vi "gradient_ascent_test.vi"() -> ()   [LabVIEW 2024]
uses:
  <vilib>/numeric/Random Number (Range) DBL.vi
panel:
  in  "N trials":dbl=16.0
  out "diff":dbl
  out "XY Graph 2":cluster{dbl[], dbl[]}[](graph)
  out "end result":dbl
  in  "k":dbl=150.0
  out "start X":dbl=75.0
  out "StdDev":dbl
  out "Mean":dbl
  # "Used only to create Gaussian to optimize"
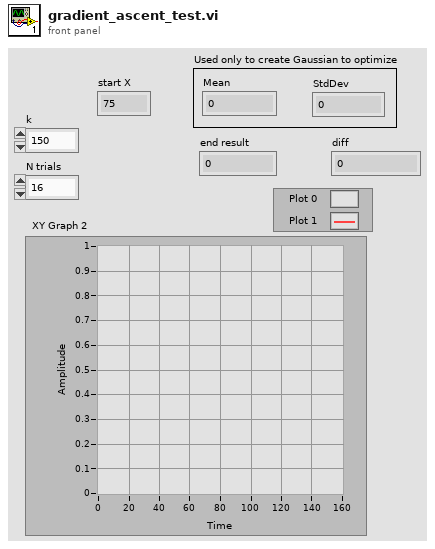
[diagram p1: front panel]
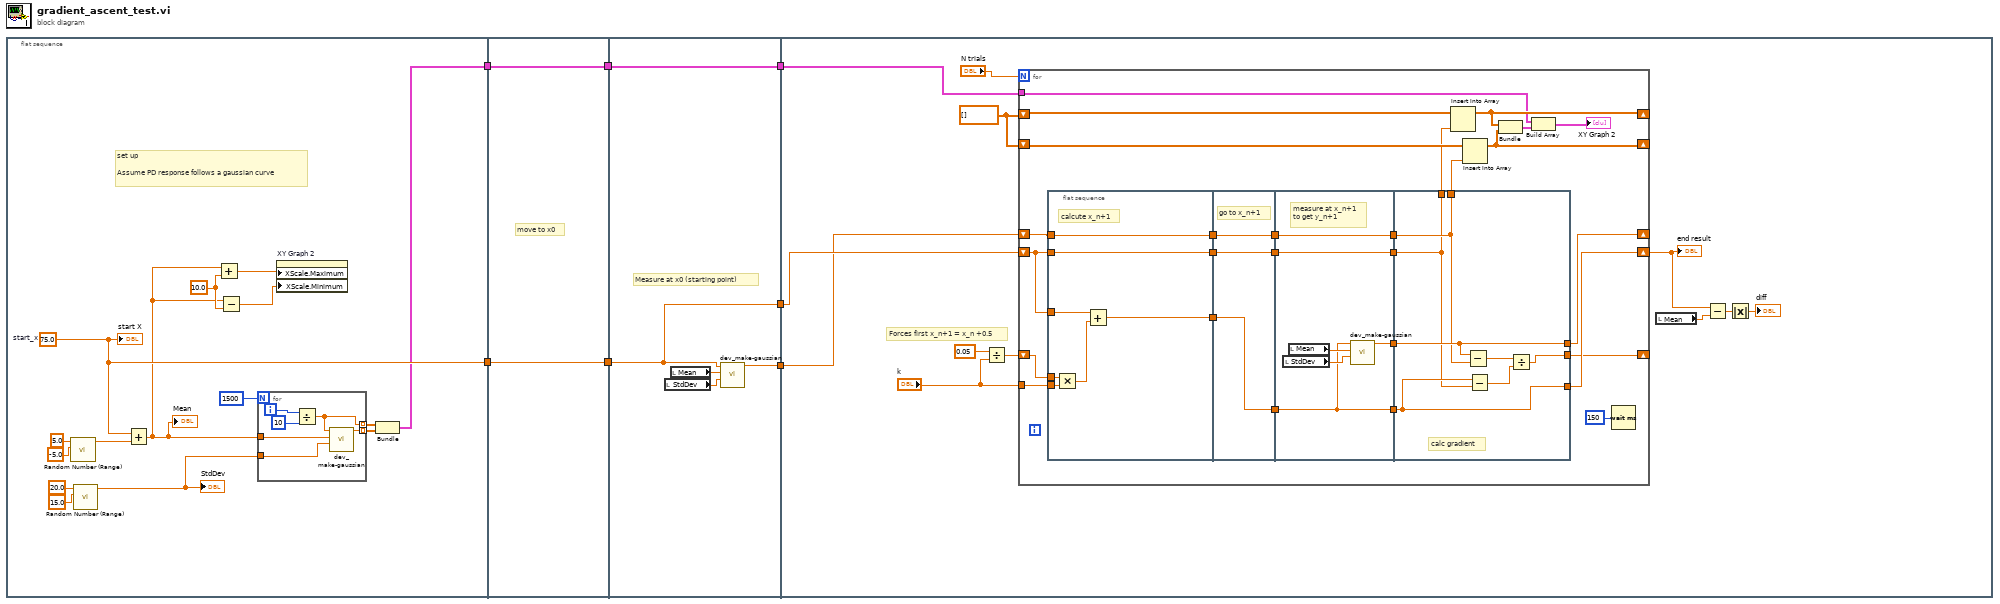
[diagram p0: block diagram]
diagram:
  n1 = flat-sequence {
    tunnel: [w13] -> w7
    tunnel: [w12] -> w1
    tunnel: w7 -> [w30]
    tunnel: [w30] -> w6
    tunnel: [w29] -> w2
    tunnel: w1 -> [w29]
    tunnel: w6 -> [w32]
    tunnel: [w33] -> w5
    tunnel: [w32] -> w4
    tunnel: [w31] -> w3
    tunnel: w2 -> [w31]
    tunnel: w5 -> [w46]
    tunnel: w4 -> [w47]
    tunnel: w3 -> [w40]
    frame #0 {
      w9 = 10.0 ("y")
      w13 = 75.0  # start_x
      # "set up\n\nAssume PD response follows a gaussian curve"
      n2 = call-poly <vilib>:"Random Number (Range).vi"("lower bound (0)"=-5.0, "upper bound (100)"=5.0) -> ("number"=w14:dbl)  [unwired: 9 in]
      n3 = call-poly <vilib>:"Random Number (Range).vi"("lower bound (0)"=15.0, "upper bound (100)"=20.0) -> ("number"=w20:dbl)  [unwired: 9 in]
      "StdDev" <- w20
      n4 = Add(x=w13, y=w14) -> (x+y=w8:dbl)
      "Mean" <- w8
      n5 = Add(x=w8, y=w9) -> (x+y=w11:dbl)
      n6 = Subtract(x=w8, y=w9) -> (x-y=w10:dbl)
      n7 = for {
        N: 1500 -> [_]
        tunnel: w20 -> [w28]
        tunnel: [w27] -> w18 mode=indexing
        tunnel: [w24] -> w17 mode=indexing
        tunnel: w8 -> [w26]
        i -> [w25]
        n8 = Divide(x=w25, y=10) -> (x/y=w24:dbl)
        n9 = call "dev_make-gaussian.vi"("StdDev"=w28, "Mean"=w26, "in"=w24) -> ("out"=w27:dbl)  [unwired: 8 in]
      }
      n10 = property on="XY Graph 2" class="XYGraph (strict)"("XScale.Maximum"=w11, "XScale.Minimum"=w10) -> ()  [unwired: 2 in, 2 out]
      n11 = Bundle(w17, w18) -> (w12:cluster{dbl[], dbl[]})  [unwired: 1 in]
      "start X" <- w13
    }
    frame #1 {
      # "move to x0"
    }
    frame #2 {
      # "Measure at x0 (starting point)"
      n12 = local read "StdDev"() -> (w34:dbl)
      n13 = local read "Mean"() -> (w35:dbl)
      n14 = call "dev_make-gaussian.vi"("StdDev"=w34, "Mean"=w35, "in"=w32) -> ("out"=w33:dbl)  [unwired: 8 in]
    }
    frame #3 {
      w41 = dbl[] []
      # "Forces first x_n+1 = x_n +0.5"
      n15 = Divide(x=0.05, y="k") -> (x/y=w37:dbl)
      n16 = for {
        N: "N trials" -> [_]
        shift-right: [w63] -> _
        shift-left: w37 -> [w74]
        shift-right: [w70] -> w45
        shift-left: w47 -> [w53]
        shift-right: [w67] -> _
        shift-left: w46 -> [w54]
        tunnel: "k" -> [w73]
        shift-right: [w59] -> _
        shift-left: w41 -> [w61]
        shift-right: [w58] -> _
        shift-left: w41 -> [w60]
        tunnel: w40 -> [w57]
        n17 = flat-sequence {
          tunnel: w74 -> [w81]
          tunnel: w73 -> [w80]
          tunnel: w53 -> [w77]
          tunnel: [w79] -> w72
          tunnel: w54 -> [w78]
          tunnel: [w78] -> w66
          tunnel: w53 -> [w76]
          tunnel: [w76] -> w51
          tunnel: w72 -> [w84]
          tunnel: [w84] -> w71
          tunnel: w66 -> [w83]
          tunnel: [w83] -> w65
          tunnel: [w82] -> w52
          tunnel: w51 -> [w82]
          tunnel: w71 -> [w88]
          tunnel: [w88] -> w69
          tunnel: [w87] -> w68
          tunnel: w65 -> [w86]
          tunnel: [w86] -> w64
          tunnel: w52 -> [w85]
          tunnel: [w85] -> w50
          tunnel: [w92] -> w70
          tunnel: w69 -> [w92]
          tunnel: w68 -> [w94]
          tunnel: [w94] -> w67
          tunnel: w64 -> [w93]
          tunnel: [w95] -> w63
          tunnel: w50 -> [w91]
          tunnel: [w93] -> w49
          tunnel: [w91] -> w48
          frame #0 {
            # "calcute x_n+1"
            n18 = Multiply(x=w81, y=w80) -> (x*y=w75:dbl)
            n19 = Add(x=w77, y=w75) -> (x+y=w79:dbl)
          }
          frame #1 {
            # "go to x_n+1"
          }
          frame #2 {
            # "measure at x_n+1\nto get y_n+1"
            n20 = local read "StdDev"() -> (w89:dbl)
            n21 = local read "Mean"() -> (w90:dbl)
            n22 = call "dev_make-gaussian.vi"("StdDev"=w89, "Mean"=w90, "in"=w88) -> ("out"=w87:dbl)  [unwired: 8 in]
          }
          frame #3 {
            # "calc gradient"
            n23 = Subtract(x=w94, y=w93) -> (x-y=w97:dbl)
            n24 = Subtract(x=w92, y=w91) -> (x-y=w96:dbl)
            n25 = Divide(x=w97, y=w96) -> (x/y=w95:dbl)
          }
        }
        n26 = Insert Into Array(array=w61, new element=w48) -> (w59:dbl[])  [unwired: 1 in]
        n27 = Insert Into Array(array=w60, new element=w49) -> (w58:dbl[])  [unwired: 1 in]
        n28 = Bundle(w59, w58) -> (w56:cluster{dbl[], dbl[]})  [unwired: 1 in]
        n29 = Build Array(w57, w56) -> (→"XY Graph 2":cluster{dbl[], dbl[]}[])
        n30 = Wait (ms)(milliseconds to wait=u32 150) -> ()  [unwired: 1 out]
      }
      "end result" <- w45
      n31 = local read "Mean"() -> (w44:dbl)
      n32 = Subtract(x=w45, y=w44) -> (x-y=w43:dbl)
      n33 = Absolute Value(x=w43) -> (abs(x)=→"diff":dbl)
    }
  }
